vi "Compensation(SubVI).vi"(11 "Array in":waveform(dbl)[](array[waveform])) -> (3 "Array out":waveform(dbl)[](array[waveform]))   [LabVIEW 2012]
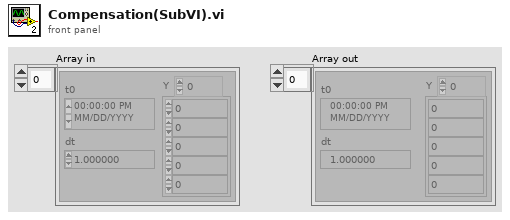
[diagram p1: front panel]
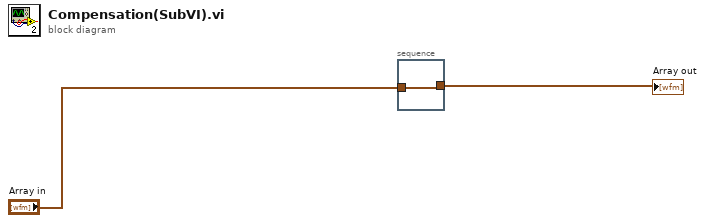
[diagram p0: block diagram]
diagram:
  n1 = stacked-sequence {
    tunnel: "Array in" -> [w3]
    tunnel: [w3] -> w2
    frame #0 {
    }
  }
  "Array out" <- w2
